vi "VI Import.vi"(6 "Drop Position (0, 0)":cluster{"Left":i32, "Top":i32}, 7 "Application Refnum":refnum<vi>, 8 "error in (no error)":errorcluster, 9 "Copy to (\"VI\")":enum8{"VI", "Clipboard"}(ring), 10 "VI Path (.vi)":path, 11 "VI Refnum in (NaN=New VI)":refnum<vi>) -> (0 "error out":errorcluster, 2 "Created New VI?":bool, 3 "VI Refnum out":refnum<vi>)   [LabVIEW 2022 SP3, in "VI-Snippet.lvlib"]
doc: "Import a VI Snippet from the <b>VI Snippet Path (*.png)</b>. Set <b>Copy to</b> as either <b>\"VI\"</b> or <b>\"Clipboard\"</b> to copy the VI Snippet content to a existing/new VI (<b>VI Refnum/NaN</b>) or copy the content to the clipboard. By default, this copies the VI Snippet to a new VI. Specify the <b>Drop Position</b> when placing content into an existing VI. The <b>Drop Position</b> has no effect for new VIs. <b>Copy to</b> <b>\"Clipboard\"</b> does not return a <b>VI Refnum out</b>."
uses:
  VI-Snippet.lvlib
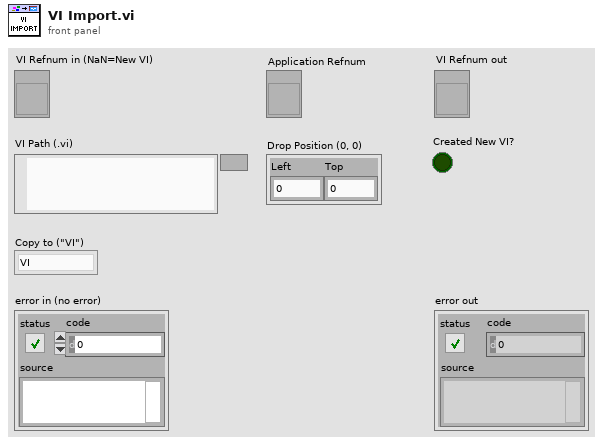
[diagram p1: front panel]
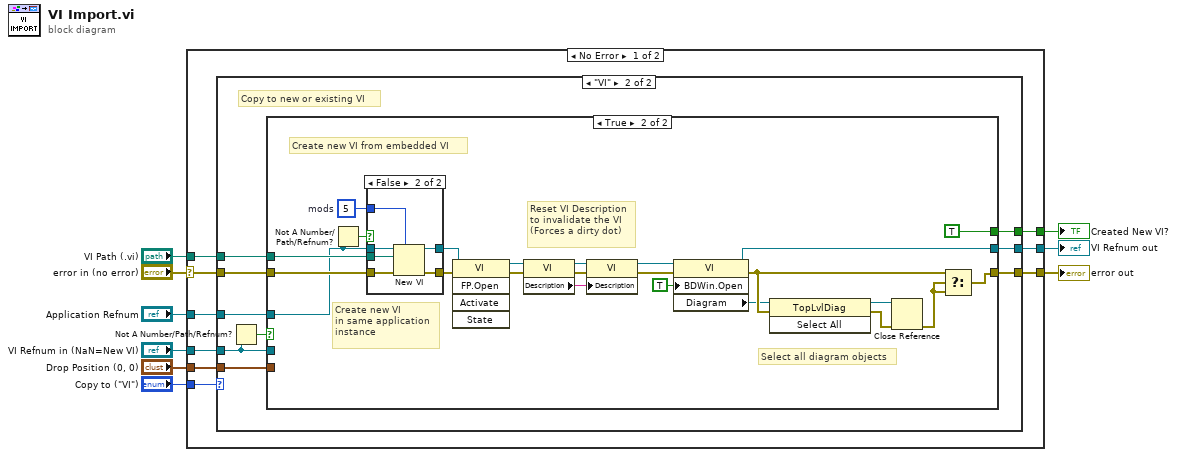
[diagram p0: block diagram]
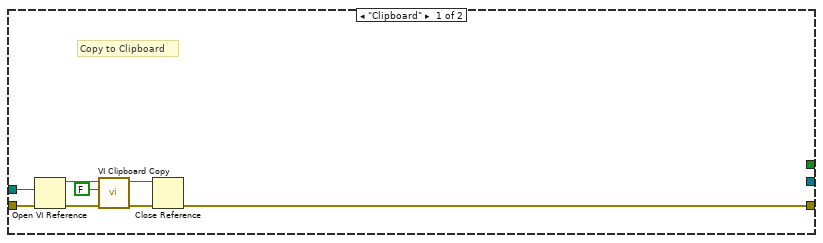
[diagram p2: hidden frame]
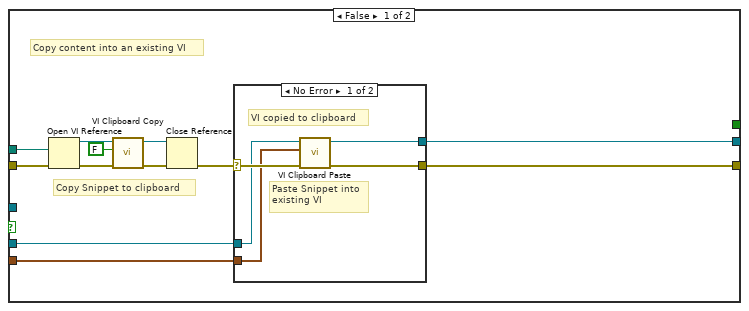
[diagram p3: hidden frame]
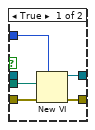
[diagram p5: hidden frame]
diagram:
  n1 = case shown="No Error" "error in (no error)" {
    selector: "error in (no error)" -> [w12 w90]
    tunnel: "VI Path (.vi)" -> [w11 _]
    tunnel: "VI Refnum in (NaN=New VI)" -> [w13 w89]
    tunnel: "Drop Position (0, 0)" -> [w18 _]
    tunnel: [w10 w90] -> w8
    tunnel: [w17 w89] -> w6
    tunnel: [w16 _] -> w5
    tunnel: "Copy to (\"VI\")" -> [w15 _]
    tunnel: "Application Refnum" -> [w14 _]
    frame No Error {
      n2 = case shown="\"VI\"" w15 {
        tunnel: w18 -> [_ w35]
        tunnel: [_ w34] -> w17
        tunnel: [_ w33] -> w16
        tunnel: w12 -> [w21 w32]
        tunnel: w13 -> [_ w31]
        tunnel: [w19 w29] -> w10
        tunnel: w11 -> [w20 w28]
        tunnel: w14 -> [_ w27]
        frame "Clipboard" {
          # "Copy to Clipboard"
          n3 = Open VI Reference(vi path=w20, error in (no error)=w21) -> (vi reference=w24:refnum<vi>, error out=w25:errorcluster)  [unwired: 4 in]
          n4 = call "VI Clipboard Copy.vi"("error in (no error)"=w25, "Selection List Only? (F=All)"=FALSE ("Selected GObjects Only? (F)"), "VI Refnum in"=w24) -> ("error out"=w26:errorcluster, "dup VI Refnum"=w23:refnum<vi>)  [unwired: 7 in]
          n5 = Close Reference(reference=w23, error in (no error)=w26) -> (error out=w19:errorcluster)
        }
        frame "VI" {
          # "Copy to new or existing VI"
          n6 = Not A Number/Path/Refnum?(number/path/refnum=w31) -> (NaN/Path/Refnum?=w30:bool)
          n7 = case shown="True" w30 {
            tunnel: w31 -> [w47 _]
            tunnel: w35 -> [w46 _]
            tunnel: [w45 w68] -> w29
            tunnel: [w44 w61] -> w34
            tunnel: [_ TRUE ("New VI?")] -> w33
            tunnel: w32 -> [w43 w77]
            tunnel: w28 -> [w37 w72]
            tunnel: w27 -> [_ w65]
            frame False {
              # "Copy content into an existing VI"
              # "Copy Snippet to clipboard"
              n8 = Open VI Reference(vi path=w37, error in (no error)=w43) -> (vi reference=w40:refnum<vi>, error out=w41:errorcluster)  [unwired: 4 in]
              n9 = call "VI Clipboard Copy.vi"("error in (no error)"=w41, "Selection List Only? (F=All)"=FALSE ("Selected GObjects Only? (F)"), "VI Refnum in"=w40) -> ("error out"=w42:errorcluster, "dup VI Refnum"=w39:refnum<vi>)  [unwired: 7 in]
              n10 = Close Reference(reference=w39, error in (no error)=w42) -> (error out=w36:errorcluster)
              n11 = case shown="No Error" w36 {
                selector: w36 -> [w52 w54]
                tunnel: w47 -> [w49 w53]
                tunnel: w46 -> [w48 _]
                tunnel: [w51 w54] -> w45
                tunnel: [w50 w53] -> w44
                frame No Error {
                  # "VI copied to clipboard"
                  # "Paste Snippet into\nexisting VI"
                  n12 = call "VI Clipboard Paste.vi"("error in (no error)"=w52, "Drop Position (0, 0)"=w48, "VI Refnum in"=w49) -> ("error out"=w51:errorcluster, "VI Refnum out"=w50:refnum<vi>)  [unwired: 7 in]
                }
                frame Error {
                  # "Failed to copy \nVI Snippet to clipboard"
                }
              }
            }
            frame True {
              w63 = u32 5  # mods
              # "Reset VI Description\nto invalidate the VI\n(Forces a dirty dot)"
              # "Select all diagram objects"
              # "Create new VI\nin same application\ninstance"
              # "Create new VI from embedded VI"
              n13 = Not A Number/Path/Refnum?(number/path/refnum=w65) -> (NaN/Path/Refnum?=w64:bool)
              n14 = case shown="False" w64 {
                tunnel: w77 -> [w82 w88]
                tunnel: [w81 w87] -> w76
                tunnel: [w80 w86] -> w62
                tunnel: w72 -> [w79 w85]
                tunnel: w65 -> [_ w84]
                tunnel: w63 -> [w78 w83]
                frame True {
                  n15 = New VI(7:w78, 8:w82, 10:w79) -> (0:w81:errorcluster, 3:w80:refnum<vi>)  [unwired: 4 in]
                }
                frame False {
                  n16 = New VI(7:w83, 8:w88, 10:w85, 11:w84) -> (0:w87:errorcluster, 3:w86:refnum<vi>)  [unwired: 3 in]
                }
              }
              n17 = invoke class="VI" method="FP.Open"(reference=w62, error in=w76) -> (reference out=w75:refnum<vi>, error out=w60:errorcluster)  [unwired: 3 in, 3 out]
              n18 = property class="VI"(reference=w75, error in=w60) -> (reference out=w59:refnum<vi>, error out=w58:errorcluster, "Description"=w55:string)
              n19 = property class="VI"(reference=w59, error in=w58, "Description"=w55) -> (reference out=w56:refnum<vi>, error out=w57:errorcluster)
              n20 = property class="VI"(reference=w56, error in=w57, "BDWin.Open"=TRUE ("Block Diagram Window:Open")) -> (reference out=w61:refnum<vi>, error out=w67:errorcluster, "Diagram"=w66:refnum<vi>)
              n21 = invoke class="TopLvlDiag" method="Select All"(reference=w66, error in=w67) -> (reference out=w71:refnum<vi>, error out=w70:errorcluster)  [unwired: 1 in, 1 out]
              n22 = Close Reference(reference=w71, error in (no error)=w70) -> (error out=w69:errorcluster)
              n23 = Select(t=w67, s=w69, f=w69) -> (s? t:f=w68:errorcluster)
            }
          }
        }
      }
    }
    frame Error {
    }
  }
  "error out" <- w8
  "VI Refnum out" <- w6
  "Created New VI?" <- w5
